vi "bundler.vi"(10 "scalar":dbl=1000.0, 11 "input ticks":i32[](array[numeric])=[1, 1]) -> (3 "output tick cluster":cluster{"high ticks":i32, "low ticks":i32})   [LabVIEW 2019]
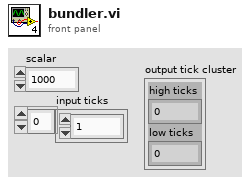
[diagram p1: front panel]
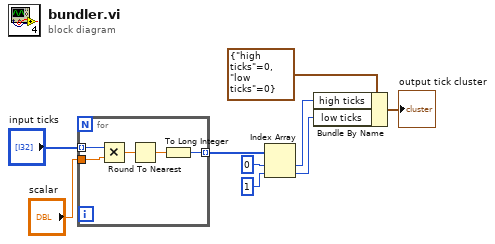
[diagram p0: block diagram]
diagram:
  n1 = for {
    tunnel: "input ticks" -> [w14] mode=indexing
    tunnel: "scalar" -> [w13]
    tunnel: [w10] -> w2 mode=indexing
    n2 = Multiply(x=w14, y=w13) -> (x*y=w12:dbl)
    n3 = Round To Nearest(number=w12) -> (nearest integer value=w11:dbl)
    n4 = To Long Integer(number=w11) -> (32bit integer=w10:i32)
  }
  n5 = Index Array(array=w2, index #1=0 ("index"), index #2=1 ("index")) -> (element #1=w6:i32, element #2=w5:i32)
  n6 = Bundle By Name(cluster=cluster{"high ticks":i32, "low ticks":i32} {"high ticks"=0, "low ticks"=0} ("input cluster"), "high ticks"=w6, "low ticks"=w5) -> (→"output tick cluster":cluster{"high ticks":i32, "low ticks":i32})
